vi "TellSelf.vi"(6 "Error":errorcluster, 7 "Actor":refnum<class "Actor.lvclass">, 9 "Payload":T6, 10 "Priority":bool, 11 "Actor":T1) -> (3 "Actor":T1, 4 "Error":errorcluster, 5 "Actor":refnum<class "Actor.lvclass">)   [LabVIEW 2020, in "_Template.lvlib" / "{{Msg}}.lvlib"]
uses:
  {{Msg}}.lvlib
  jettl/jettl/Actor/Actor.lvclass
  jettl/jettl/Metadata/Metadata.lvclass
  jettl/jettl/Msg/Msg.lvclass
  Msg/Msg.lvclass
  jettl/jettl/jettl.lvlib
  jettl/jettl/MsgExecuteType.ctl
  Payload.ctl
  jettl/jettl/Msg.ctl
  jettl/jettl/PostSetup.ctl
  jettl/jettl/PreSetup.ctl
  jettl/jettl/MsgNames.ctl
  jettl/jettl/Lifecycle.ctl
  jettl/jettl/ActorAttribs.ctl
  jettl/jettl/ChildActors.ctl
  jettl/jettl/Actor.ctl
  jettl/jettl/Origin.ctl
  jettl/jettl/MsgAttribs.ctl
panel:
  # "This front panel should not be manipulated."
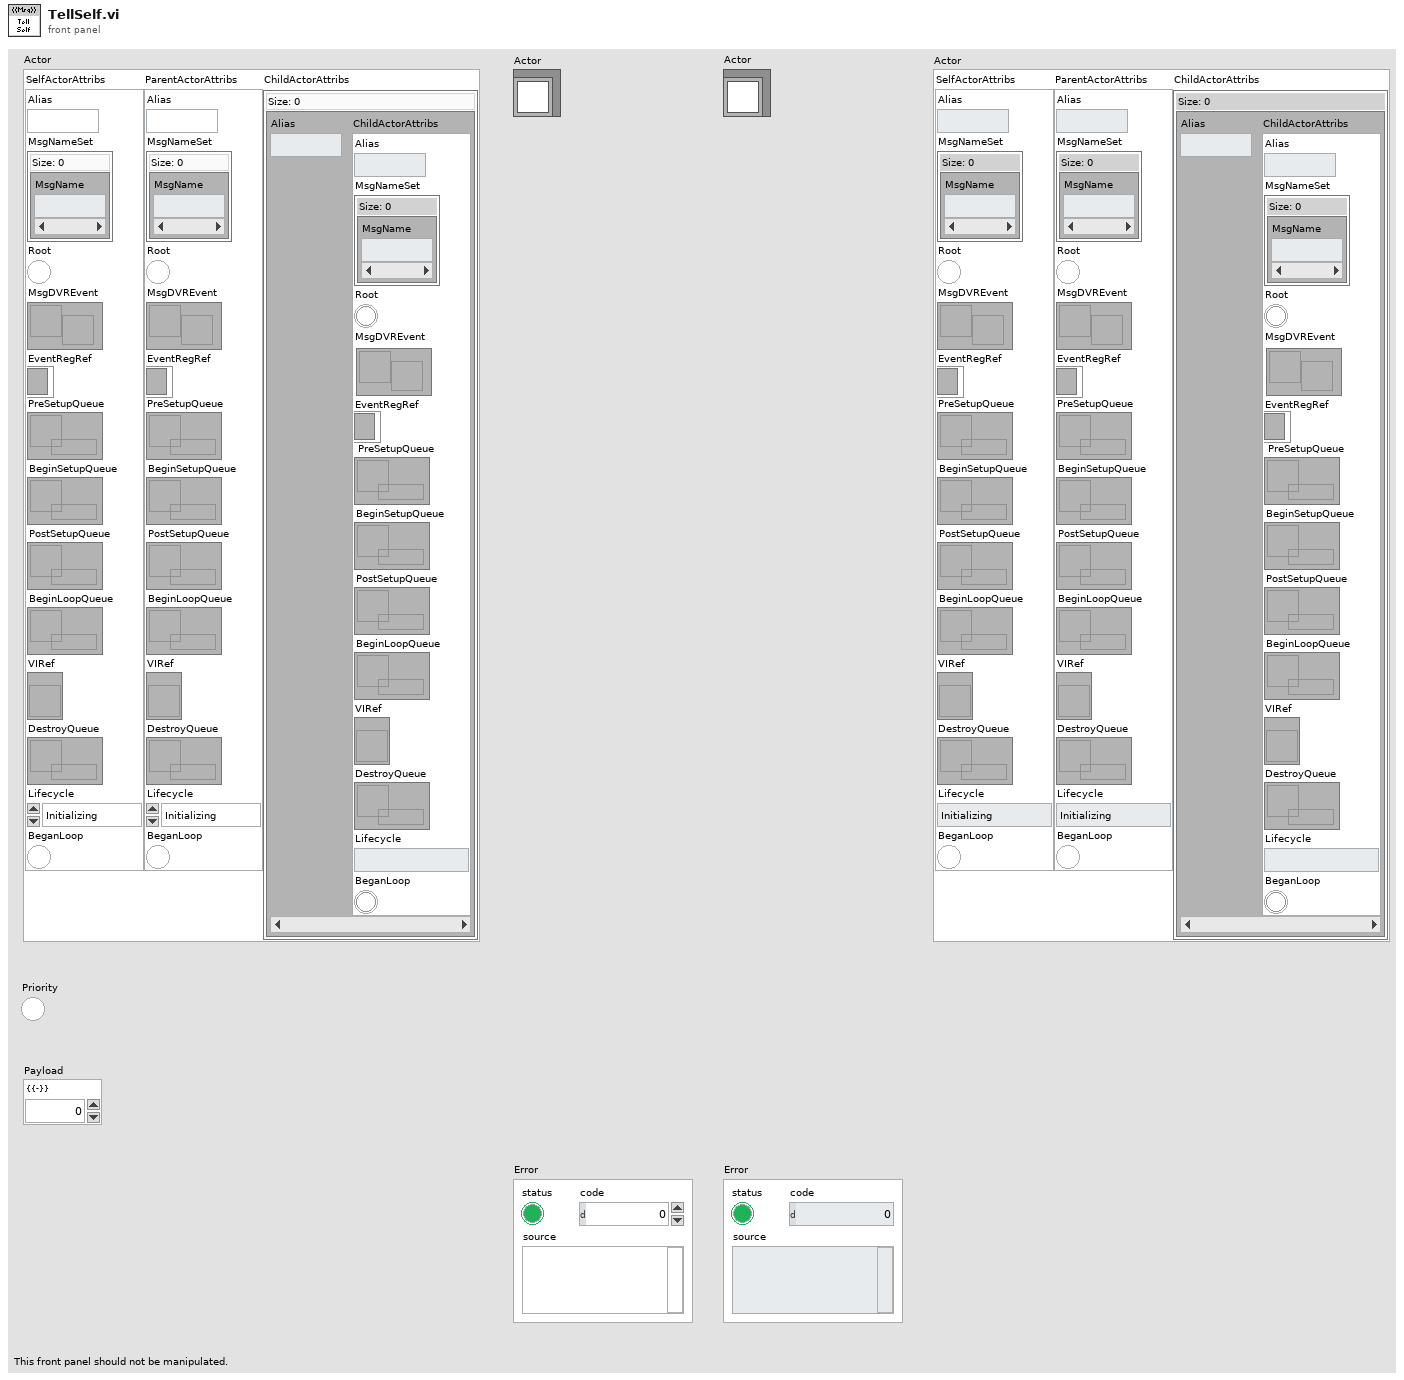
[diagram p1: front panel]
types:
  T1 = typedef "jettl.lvlib/Actor.ctl" = cluster{"SelfActorAttribs":T2, "ParentActorAttribs":T2, "ChildActorAttribs":T5}
  T2 = typedef "jettl.lvlib/ActorAttribs.ctl" = cluster{"Alias":string, "MsgNameSet":T3, "Root":bool, "MsgDVREvent":refnum<user-event>, "EventRegRef":refnum<event-registration>, "PreSetupQueue":refnum<queue>, "BeginSetupQueue":refnum<queue>, "PostSetupQueue":refnum<queue>, "BeginLoopQueue":refnum<queue>, "VIRef":refnum<vi>, "DestroyQueue":refnum<queue>, "Lifecycle":T4, "BeganLoop":bool}
  T3 = typedef "jettl.lvlib/MsgNames.ctl" = set{string}
  T4 = typedef "jettl.lvlib/Lifecycle.ctl" = enum16{"Initializing", "SettingUp", "Starting", "Running", "Stopping", "TearingDown", "Terminated"}
  T5 = typedef "jettl.lvlib/ChildActors.ctl" = map{string, T2}
  T6 = typedef "_Template.lvlib/{{Msg}}.lvlib/Payload.ctl" = cluster{"{{-}}":u8}
  T7 = typedef "jettl.lvlib/MsgExecuteType.ctl" = enum16{"Tell", "Call"}
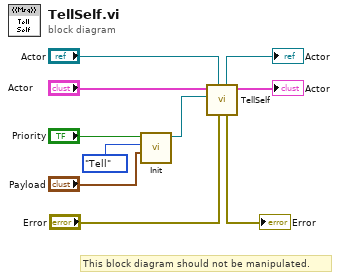
[diagram p0: block diagram]
diagram:
  # "This block diagram should not be manipulated."
  n1 = call "Init.vi"("Payload"="Payload", "MsgExecuteType"=MsgExecuteType."Tell", "Priority"="Priority") -> ("MsgDVR"=w7:refnum<data-value>)  [unwired: 8 in]
  n2 = call "TellSelf.vi"("Error"="Error", 7:"Actor"="Actor", "MsgDVR"=w7, 11:"Actor"="Actor") -> (3:"Actor"=→"Actor":T1, "Error"=→"Error":errorcluster, 5:"Actor"=→"Actor":refnum<class "Actor.lvclass">)  [unwired: 5 in]
